vi "Report Generator Unit Test.vi"() -> ()   [LabVIEW 2017]
uses:
  builds/Report Generator.lvlibp/Report Generator.lvclass
panel:
  in  "Root Path":path=path "C:/Users/Ron.Dexter.LUMINARTECH/Desktop"
  in  "Data":string[](array[string])
  in  "Data Headers":string[](array[string])
  in  "Header Data":string[](array[string])
  in  "Header Labels":string[](array[string])
  out "error out":errorcluster
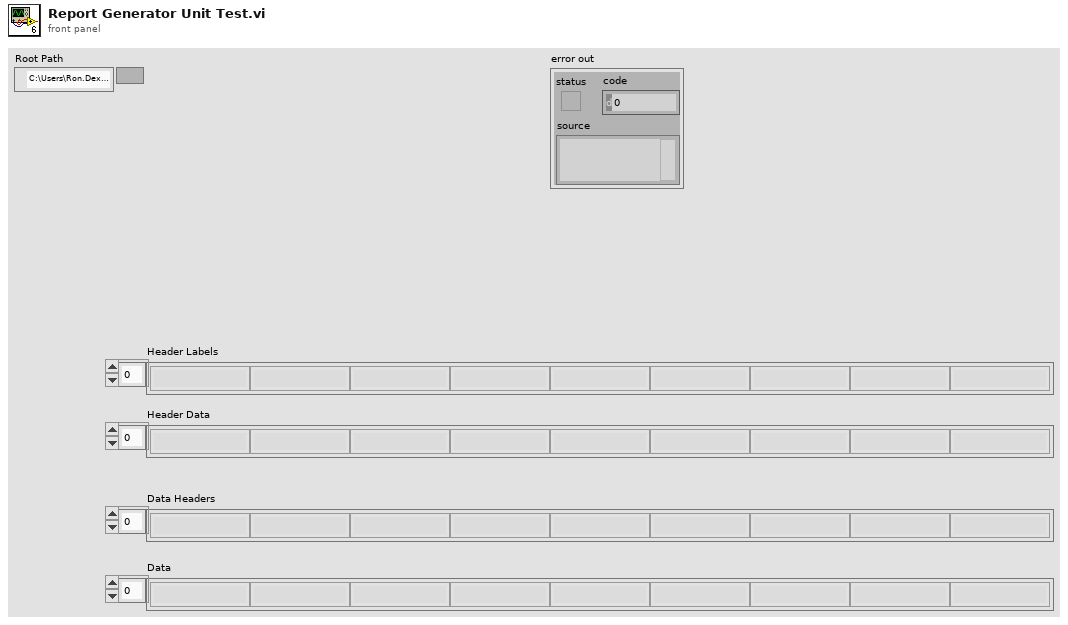
[diagram p1: front panel]
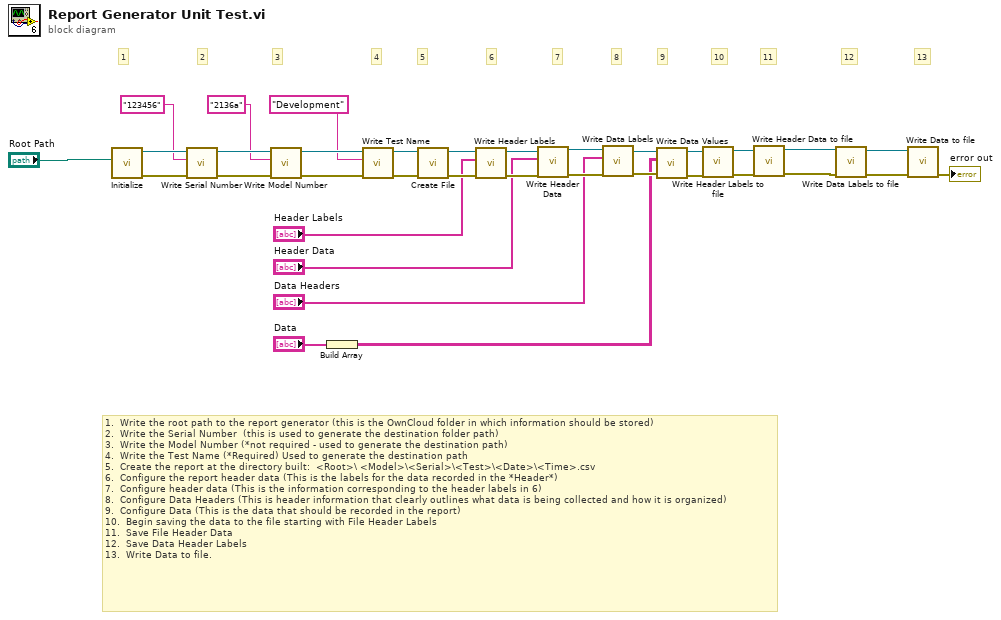
[diagram p0: block diagram]
diagram:
  # "1.  Write the root path to the report generator (this is the OwnCloud folder in which information should be stored)\n2.  Write the Serial Number  (this is used to generate the destination folder path)\n3.  Write the Model Number (*not required - used to generate the destination path)\n4.  Write the Test Name (*Required) Used to generate the destination path\n5.  Create the report at the directory built:  <Root>\\ <Model>\\<Serial>\\<Test>\\<Date>\\<Time>.csv\n6.  Configure the report header data (This is the labels for the data recorded in the *Header*)\n7.  Configure header data (This is the information corresponding to the header labels in 6)\n8.  Configure Data Headers (This is header information that clearly outlines what data is being collected and how it is organized)\n9.  Configure Data (This is the data that should be recorded in the report)\n10.  Begin saving the data to the file starting with File Header Labels\n11.  Save File Header Data\n12.  Save Data Header Labels\n13.  Write Data to file."
  # "13"
  # "12"
  # "11"
  # "10"
  # "9"
  # "8"
  # "7"
  # "6"
  # "5"
  # "4"
  # "3"
  # "2"
  # "1"
  n1 = call "Initialize.vi"("Root Path"="Root Path") -> ("error out"=w31:errorcluster, "Report Generator out"=w34:refnum<class "Report Generator.lvclass">)  [unwired: 9 in]
  n2 = call "Write Serial Number.vi"("error in (no error)"=w31, "Serial Number"="123456", "Report Generator in"=w34) -> ("error out"=w30:errorcluster, "Report Generator out"=w33:refnum<class "Report Generator.lvclass">)  [unwired: 7 in]
  n3 = call "Write Model Number.vi"("error in (no error)"=w30, "Model Number"="2136a", "Report Generator in"=w33) -> ("error out"=w29:errorcluster, "Report Generator out"=w32:refnum<class "Report Generator.lvclass">)  [unwired: 7 in]
  n4 = Build Array("Data") -> (w10:string[][])
  n5 = call "Write Test Name.vi"("error in (no error)"=w29, "Test Name"="Development", "Report Generator in"=w32) -> ("error out"=w23:errorcluster, "Report Generator out"=w24:refnum<class "Report Generator.lvclass">)  [unwired: 7 in]
  n6 = call "Create File.vi"("error in"=w23, "Report Generator in"=w24) -> ("error out"=w21:errorcluster, "Report Generator out"=w22:refnum<class "Report Generator.lvclass">)  [unwired: 8 in]
  n7 = call "Write Header Labels.vi"("error in (no error)"=w21, "Header Labels"="Header Labels", "Report Generator in"=w22) -> ("error out"=w19:errorcluster, "Report Generator out"=w18:refnum<class "Report Generator.lvclass">)  [unwired: 7 in]
  n8 = call "Write Header Data.vi"("error in (no error)"=w19, "Header Data"="Header Data", "Report Generator in"=w18) -> ("error out"=w15:errorcluster, "Report Generator out"=w16:refnum<class "Report Generator.lvclass">)  [unwired: 7 in]
  n9 = call "Write Data Labels.vi"("error in (no error)"=w15, "Data Labels"="Data Headers", "Report Generator in"=w16) -> ("error out"=w13:errorcluster, "Report Generator out"=w12:refnum<class "Report Generator.lvclass">)  [unwired: 7 in]
  n10 = call "Write Data Values.vi"("error in (no error)"=w13, "Data Values"=w10, "Report Generator in"=w12) -> ("error out"=w9:errorcluster, "Report Generator out"=w8:refnum<class "Report Generator.lvclass">)  [unwired: 7 in]
  n11 = call "Write Header Labels to file.vi"("error in"=w9, "Report Generator in"=w8) -> ("error out"=w7:errorcluster, "Report Generator out"=w6:refnum<class "Report Generator.lvclass">)  [unwired: 8 in]
  n12 = call "Write Header Data to file.vi"("error in"=w7, "Report Generator in"=w6) -> ("error out"=w4:errorcluster, "Report Generator out"=w5:refnum<class "Report Generator.lvclass">)  [unwired: 8 in]
  n13 = call "Write Data Labels to file.vi"("error in"=w4, "Report Generator in"=w5) -> ("error out"=w2:errorcluster, "Report Generator out"=w3:refnum<class "Report Generator.lvclass">)  [unwired: 8 in]
  n14 = call "Write Data to file.vi"("error in"=w2, "Report Generator in"=w3) -> ("error out"=→"error out":errorcluster)  [unwired: 8 in, 1 out]
